vi "construct.vi"(8 "error in (no error)":errorcluster, 9 "message":string, 10 "code":dbl) -> (0 "error out":errorcluster, 3 "Child out":refnum<class "Child.lvclass">)   [LabVIEW 2021, in "Child.lvclass"]
uses:
  Child.lvclass
  Child.lvclass/Child.ctl
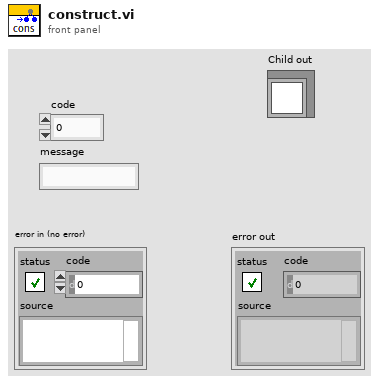
[diagram p1: front panel]
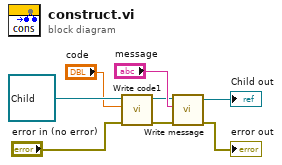
[diagram p0: block diagram]
diagram:
  n1 = call "Write code1.vi"("error in (no error)"="error in (no error)", "code1"="code", "Child in"=refnum<class "Child.lvclass"> refnum ("Child.lvclass")) -> ("error out"=w6:errorcluster, "Child out"=w3:refnum<class "Child.lvclass">)  [unwired: 7 in]
  n2 = call-dynamic "Write message.vi"("error in (no error)"=w6, "message"="message", "Child in"=w3) -> ("error out"=→"error out":errorcluster, "Child out"=→"Child out":refnum<class "Child.lvclass">)  [unwired: 7 in]
